vi "ex_Modify Signal Name.vi"(8 "error in (no error)":errorcluster, 10 "Name Modifier":string, 11 "waveform in":waveform(dbl)={"t0"=timestamp(0 s since 1904-01-01), "dt"=0.0, "Y"=[]}) -> (0 "error out":errorcluster, 3 "waveform out":waveform(dbl))   [LabVIEW 2020]
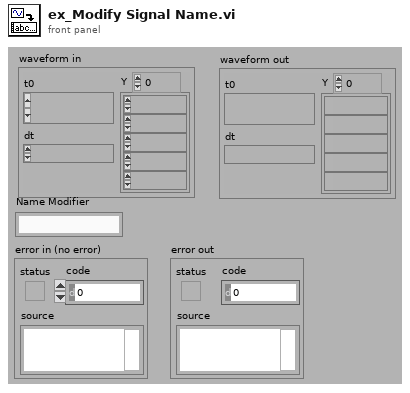
[diagram p1: front panel]
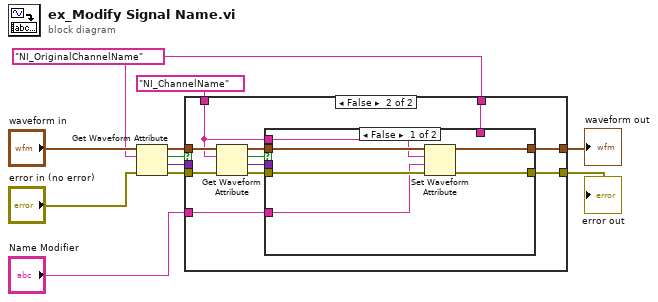
[diagram p0: block diagram]
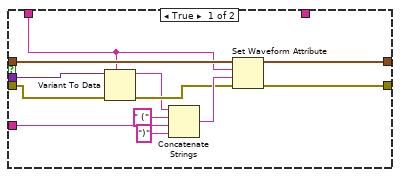
[diagram p2: hidden frame]
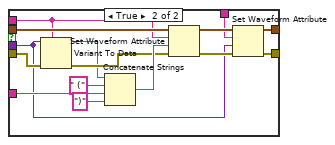
[diagram p3: hidden frame]
diagram:
  w1 = "NI_OriginalChannelName" ("name")
  n1 = Get Waveform Attribute(4:"error in (no error)", 6:w1, 7:"waveform in") -> (0:w4:errorcluster, 1:w5:variant, 2:w10:bool, 3:w11:waveform(dbl))  [unwired: 1 in]
  n2 = case shown="False" w10 {
    tunnel: w11 -> [w23 w32]
    tunnel: "Name Modifier" -> [w13 w34]
    tunnel: [w19 w27] -> w3
    tunnel: [w18 w33] -> w2
    tunnel: "NI_ChannelName" ("name") -> [w12 w28]
    tunnel: w5 -> [w17 _]
    tunnel: w4 -> [w16 w29]
    tunnel: w1 -> [_ w26]
    frame True {
      n3 = Variant To Data(error in=w16, type=w12, Variant=w17) -> (data=w14:string, error out=w15:errorcluster)
      n4 = Concatenate Strings(w14, " (" ("string"), w13, ")" ("string")) -> (w20:string)
      n5 = Set Waveform Attribute(4:w15, 5:w20, 6:w12, 7:w23) -> (0:w18:errorcluster, 3:w19:waveform(dbl))  [unwired: 1 out]
    }
    frame False {
      n6 = Get Waveform Attribute(4:w29, 6:w28, 7:w32) -> (0:w30:errorcluster, 1:w25:variant, 2:w24:bool, 3:w31:waveform(dbl))  [unwired: 1 in]
      n7 = case shown="False" w24 {
        tunnel: w34 -> [w38 w54]
        tunnel: [w35 w50] -> w33
        tunnel: w31 -> [w40 w49]
        tunnel: w30 -> [w39 w48]
        tunnel: w28 -> [w37 w46]
        tunnel: [w36 w44] -> w27
        tunnel: w26 -> [_ w43]
        tunnel: w25 -> [_ w42]
        frame False {
          n8 = Set Waveform Attribute(4:w39, 5:w38, 6:w37, 7:w40) -> (0:w35:errorcluster, 3:w36:waveform(dbl))  [unwired: 1 out]
        }
        frame True {
          n9 = Variant To Data(error in=w48, type=w46, Variant=w42) -> (data=w41:string, error out=w47:errorcluster)
          n10 = Concatenate Strings(w41, " (" ("string"), w54, ")" ("string")) -> (w51:string)
          n11 = Set Waveform Attribute(4:w47, 5:w51, 6:w46, 7:w49) -> (0:w50:errorcluster, 3:w45:waveform(dbl))  [unwired: 1 out]
          n12 = Set Waveform Attribute(5:w42, 6:w43, 7:w45) -> (3:w44:waveform(dbl))  [unwired: 1 in, 2 out]
        }
      }
    }
  }
  "waveform out" <- w3
  "error out" <- w2
